vi "Register Event(Multi).vi"(8 "error in (no error)":errorcluster, 10 "Events":T1[](array[typedef]), 11 "Resister Info":T3) -> (0 "error out":errorcluster)   [LabVIEW 2019, in "Camera Engine Event.lvlib"]
uses:
  Camera Engine Event.lvlib
  <userlib>/JUL/Event Message Module/Event Message Library/Event.ctl
  <userlib>/JUL/Event Message Module/Event Message Library/Event Data Type.ctl
  Event Type.ctl
  <userlib>/JUL/Event Message Module/Event Message Library/Event Message.lvlib
panel:
  # "Input"
  # "Output"
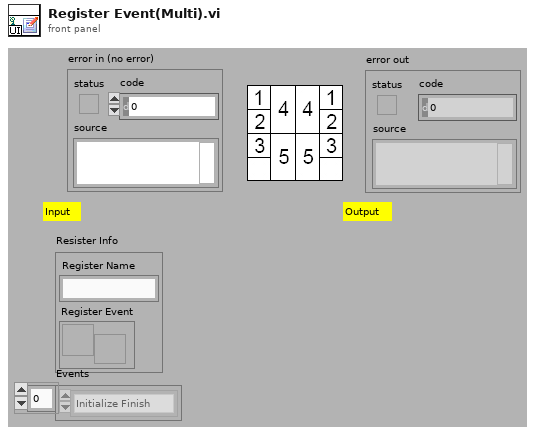
[diagram p1: front panel]
types:
  T1 = typedef "Camera Engine Event.lvlib/Event Type.ctl" = enum16{"Default", "Initialize Finish", "Button 0 Click", "Exit Click", "Exit"}
  T2 = typedef "Event Message.lvlib/Event.ctl" = refnum<user-event>
  T3 = cluster{"Register Name":string, "Register Event":T2}
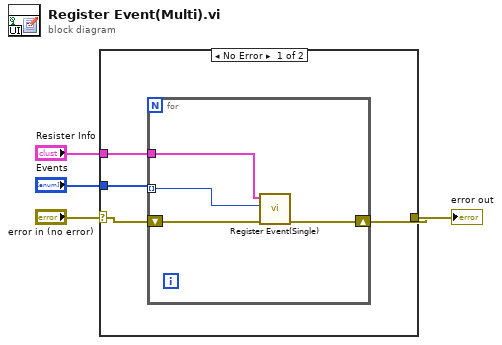
[diagram p0: block diagram]
diagram:
  n1 = case shown="No Error" "error in (no error)" {
    selector: "error in (no error)" -> [w6 w13]
    tunnel: [w5 w13] -> w2
    tunnel: "Events" -> [w8 _]
    tunnel: "Resister Info" -> [w7 _]
    frame No Error {
      n2 = for {
        tunnel: w8 -> [w11] mode=indexing
        tunnel: w7 -> [w12]
        shift-right: [w9] -> w5
        shift-left: w6 -> [w10]
        n3 = call "Register Event(Single).vi"("error in (no error)"=w10, "Event Type"=w11, "Resister Info"=w12) -> ("error out"=w9:errorcluster)  [unwired: 8 in]
      }
    }
    frame Error {
    }
  }
  "error out" <- w2
